vi "UIRef.vi"(8 "error in":errorcluster, 11 "OPC UA editor node in":refnum<class "OPC UA editor node.lvclass">) -> (0 "error out":errorcluster, 2 "VI refnum":refnum<vi>, 3 "OPC UA editor node out":refnum<class "OPC UA editor node.lvclass">)   [LabVIEW 2013, in "OPC UA editor node.lvclass"]
uses:
  OPC UA editor node.lvclass
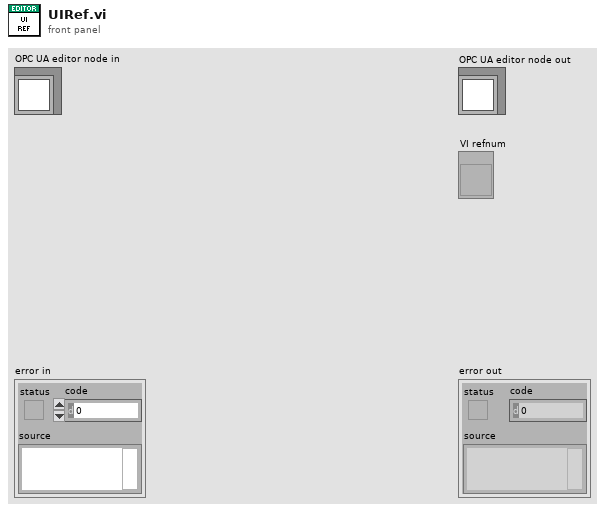
[diagram p1: front panel]
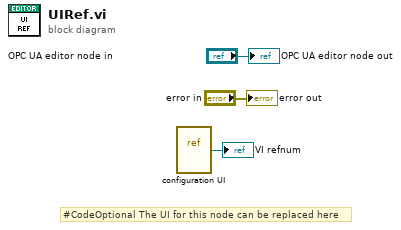
[diagram p0: block diagram]
diagram:
  # "#CodeOptional The UI for this node can be replaced here"
  n1 = vi-ref "configuration UI.vi"() -> (→"VI refnum":refnum<vi>)
  "error out" <- "error in"
  "OPC UA editor node out" <- "OPC UA editor node in"
